vi "系统设置.vi"() -> ()   [LabVIEW 2016]
uses:
  <vilib>/Utility/miscctls.llb/LVPointTypeDef.ctl
  <userlib>/_SmartBalloon/Balloon Generic/Aesthetics.ctl
  <userlib>/_SmartBalloon/Balloon/Text Balloon.lvclass
  C:/Program Files (x86)/National Instruments/LabVIEW 2016/user.lib/_SmartBalloon/Balloon Generic/Balloon.lvclass
  <userlib>/_SmartBalloon/Balloon/Init Balloon.vi
  <vilib>/ptbypt/NI_PtbyPt.lvlib
  <vilib>/Utility/config.llb/NI_LVConfig.lvlib
  PLC/PLC.lvlib
  API/WxMessage/wxpusher.lvlib
  <userlib>/_SmartBalloon/API/SmartBalloon Library.lvclass
  <userlib>/_SmartBalloon/Balloon Generic/Balloon.lvclass
panel:
  in  "站点信息设置":bool
  in  "微信关注设置":bool
  in  "自动运行启动参数":T1
  out "一级权限":bool
  in  "定时重启配置":bool
  in  "模块启用配置":bool
  in  "短信报警设置":bool
  in  "首页显示设置":bool
  in  "跨度核查":bool
  in  "空白核查":bool
  out "选项卡控件":enum32{"自由设定", "国标协议", "流量设定"}(tab)
  in  "24H周期设置":bool[](xcontrol)
  in  "多参数运行间隔":i16=4 min=1 max=24
  in  "湿化学运行间隔":i16=4 min=1 max=24
  in  "流量阈值":dbl=4.0 min=1.0 max=24.0
  in  "时间阈值":u16=4 min=1 max=24
  in  "周期设置":enum16{"自由设定", "国标协议", "流量设定"}(ring)
  out "二级权限":bool
  in  "质控启动日期":string(combo)="关闭"
  in  "跨度核查时间":u16(ring)=6 items=["00H", "01H", "02H", "03H", "04H", "05H", "06H", "07H", "08H", "09H", "10H", "11H", "12H", "13H", "14H", "15H", "16H", "17H", "18H", "19H", "20H", "21H", "22H", "23H", "关闭"]
  in  "空白核查时间":u16(ring)=2 items=["00H", "01H", "02H", "03H", "04H", "05H", "06H", "07H", "08H", "09H", "10H", "11H", "12H", "13H", "14H", "15H", "16H", "17H", "18H", "19H", "20H", "21H", "22H", "23H", "关闭"]
  in  "输入密码":u32
  out "布尔":bool
  in  "副屏显示设置":bool
  in  "开机启动":bool caption="氨氮禁用"
  in  "运行模式":enum16{"维护模式", "常规模式", "应急模式", "质控模式"}(ring)
  # "注：周期设置分为自由设定和国标协议两种。\n1：选择自由设定情况下：运行间隔将不可选用并变灰色，周期设置可自由手动勾选\n2：选择国标协议情况下：周期时间将由运行间隔选择的时间决定，下方周期设置被禁用并无法手动勾选。\n3：选择流量设定情况下：瞬时流量连续超过流量阈值到达时间阈值设定值，仪器将自动开启测量。"
  # "质控频次："
  # "零点核查时间："
  # "跨度核查时间："
  # "启动周期设置"
  # "m3/S"
  # "秒"
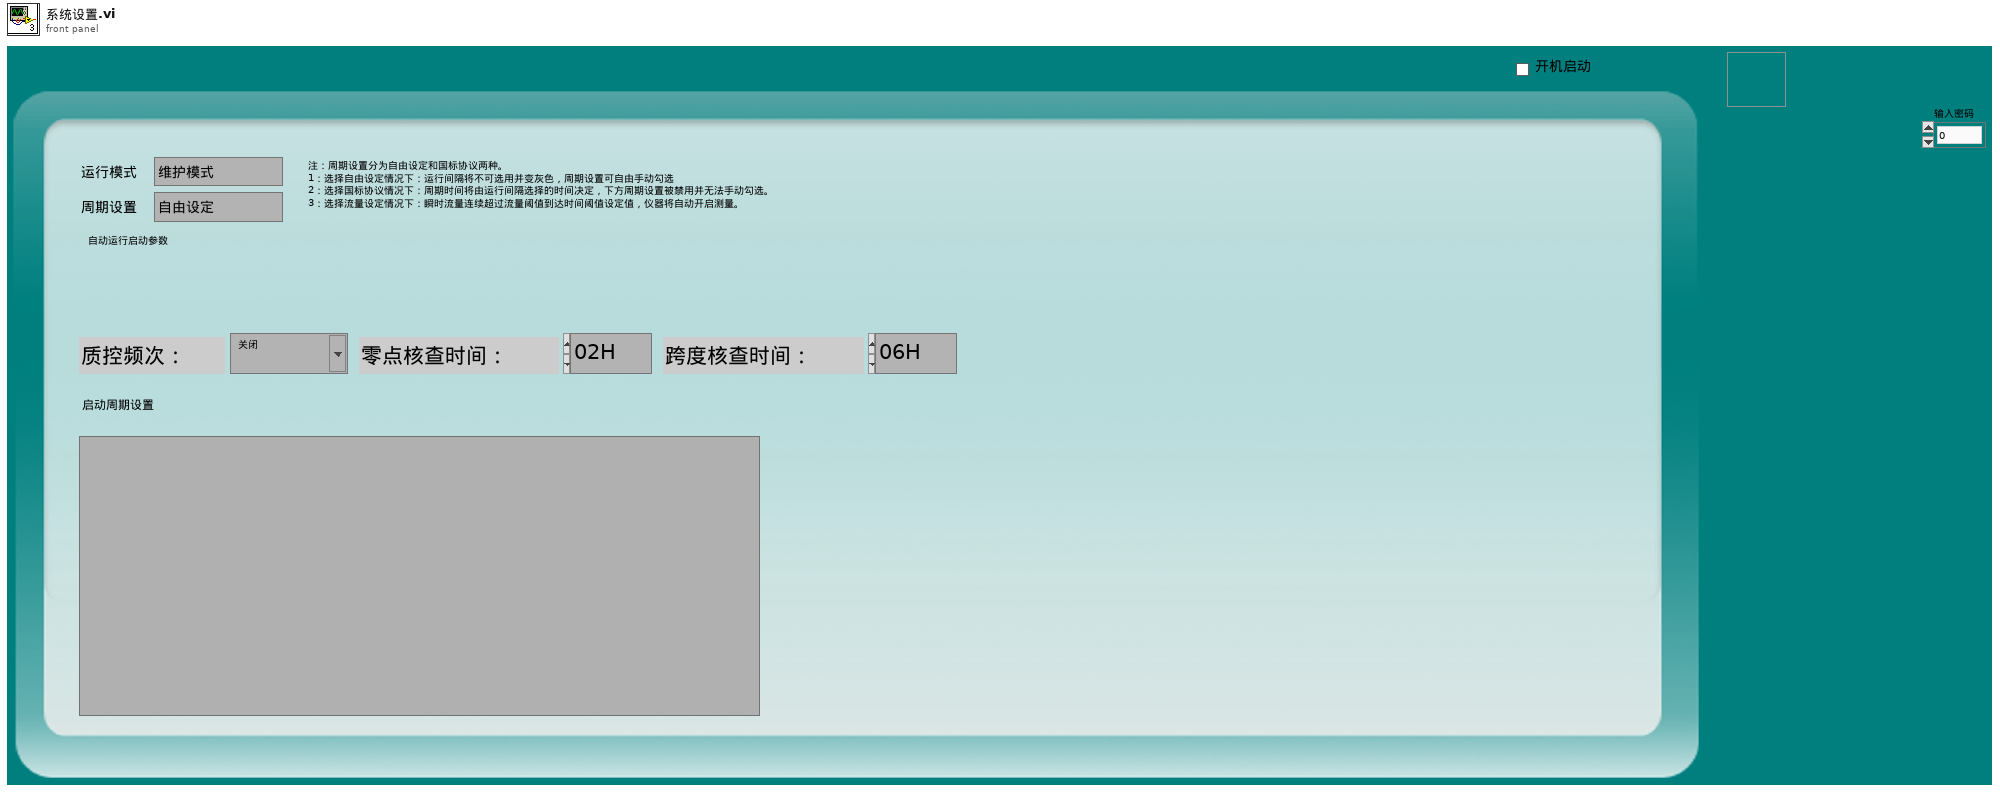
[diagram p1: front panel]
types:
  T1 = cluster{"氨氮":bool, "总磷总氮":bool, "CODmn":bool, "CODCr":bool, "多参数":bool, "超标留样启用":bool, "总氮":bool}
  T2 = typedef "LVPointTypeDef.ctl" = cluster{"Horizontal":i16, "Vertical":i16}
  T3 = cluster{"频次":enum16{"关闭", "每天", "星期一", "星期二", "星期三", "星期四", "星期五", "星期六", "星期日"}, "时":u16, "分":u16}
  T4 = typedef "LVDateTimeRec.ctl" = cluster{"秒数的小数部分":dbl, "秒":i32, "分":i32, "时":i32, "日":i32, "月":i32, "年":i32, "天数（周）":i32, "天数（年）":i32, "DST":i32}
  T5 = enum16{"关闭", "每天", "星期一", "星期二", "星期三", "星期四", "星期五", "星期六", "星期日"}
  T6 = enum32{"Bad", "Idle", "Run top level", "Running"}
  T7 = typedef "Balloon Engine.lvlib/Balloon.lvclass/Aesthetics.ctl" = cluster{"Colors":cluster{"Font Color":u32, "Panel Color":u32}, "Display Time (ms)":i32}
  T8 = typedef "NI_LVConfig.lvlib/Config Data RefNum.ctl" = refnum<k1>
  T9 = cluster{"运行模式":enum16{"维护模式", "常规模式", "应急模式", "质控模式"}}
  T10 = enum16{"启动测量", "标样核查", "零点核查", "跨度核查", "空白测试", "平行样测试", "加标回收", "空白校准", "标样校准", "初始化（清洗）", "停止测试", "仪器重启", "校时", "模式设置", "测量间隔设置"}
  T11 = cluster{"测量模式":enum16{"水样测量", "标样核查", "零点核查", "跨度核查", "空白测试", "加标回收", "平行样", "校零", "校标"}}
  T12 = cluster{"测试模式":enum16{"正常测试", "集成干预"}, "参数启用":cluster{"氨氮":bool, "总磷总氮":bool, "CODMn":bool, "CODcr":bool, "多参数":bool, "超标留样":bool, "总氮":bool}}
  T13 = cluster{"运行模式":enum16{"维护模式", "常规模式", "应急模式", "质控模式"}, "质控频次":enum16{"关闭", "每天", "星期一", "星期二", "星期三", "星期四", "星期五", "星期六", "星期日"}, "空白核查时间":u16, "跨度核查时间":u16, "24H周期设置":bool[]}
  T14 = enum32{"Invalid", "Standard", "Closed", "Hidden", "Minimized", "Maximized"}
  T15 = cluster{"氨氮":bool, "总磷总氮":bool, "CODmn":bool, "CODCr":bool, "多参数":bool, "超标留样":bool, "总氮":bool}
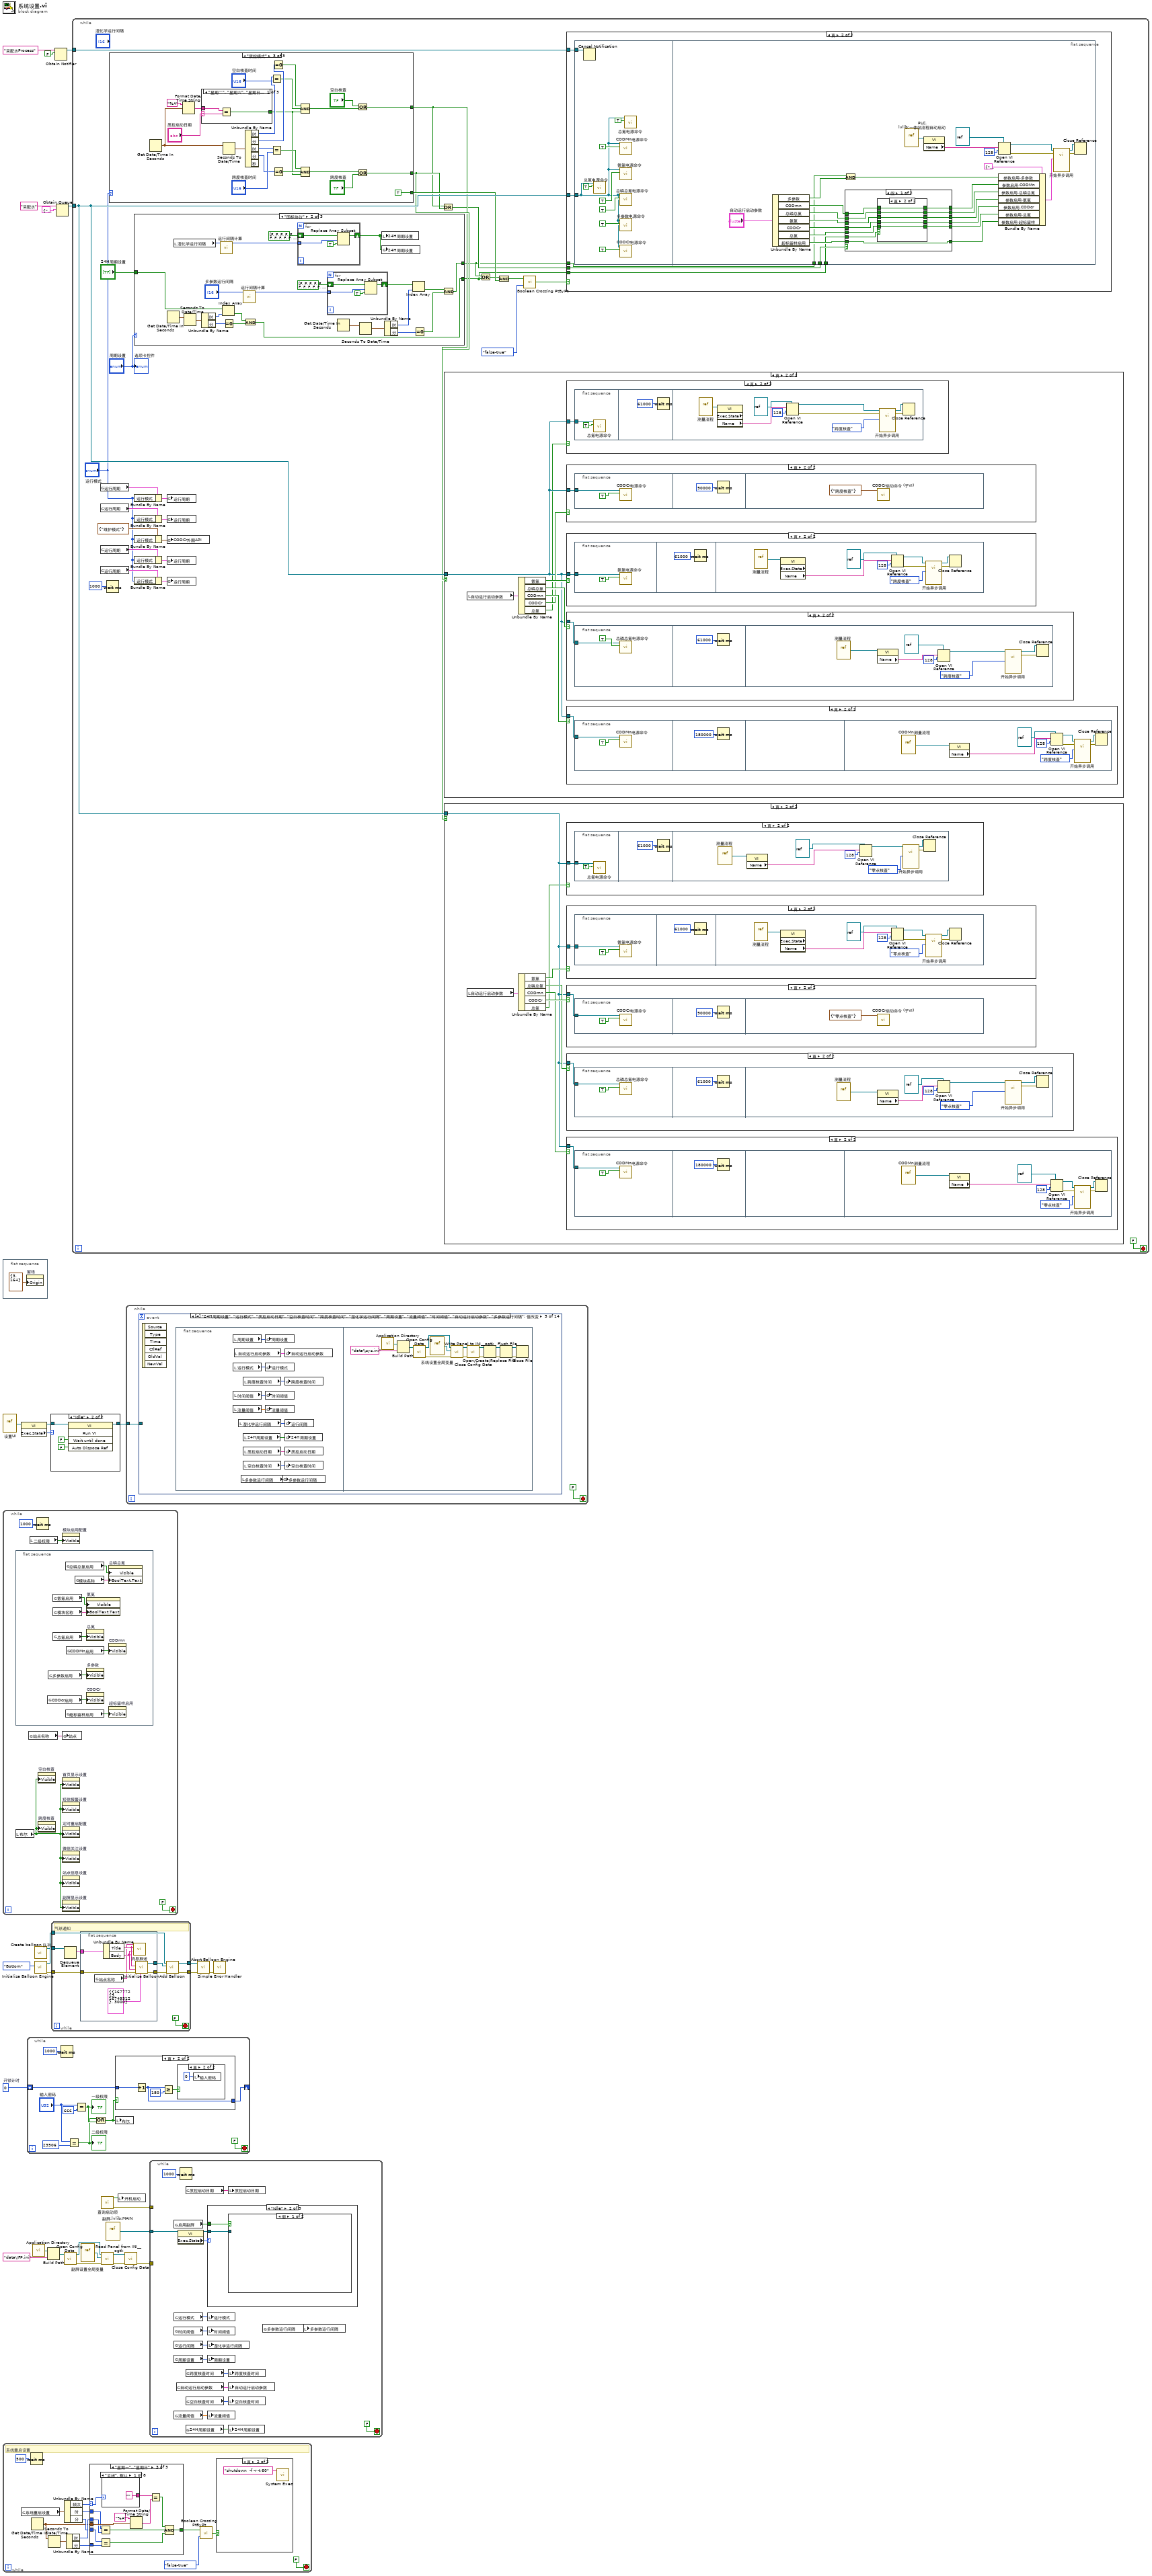
[diagram p0: block diagram]
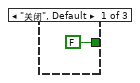
[diagram p3: hidden frame]
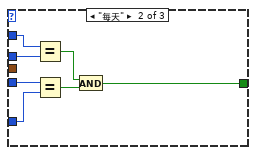
[diagram p4: hidden frame]
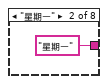
[diagram p5: hidden frame]
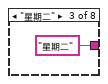
[diagram p6: hidden frame]
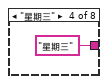
[diagram p7: hidden frame]
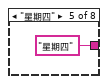
[diagram p8: hidden frame]
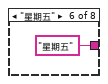
[diagram p9: hidden frame]
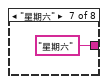
[diagram p10: hidden frame]
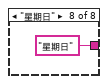
[diagram p11: hidden frame]
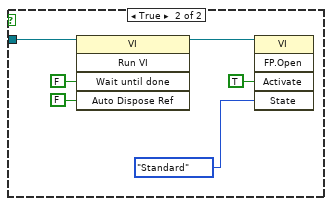
[diagram p16: hidden frame]
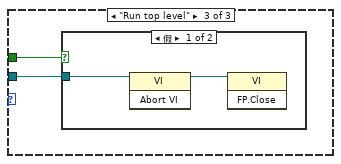
[diagram p17: hidden frame]
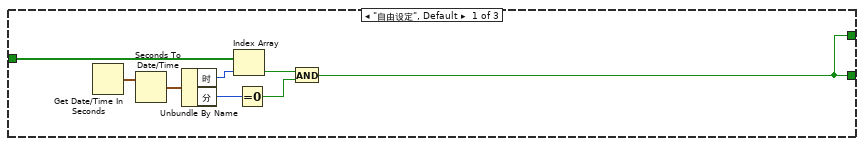
[diagram p19: hidden frame]
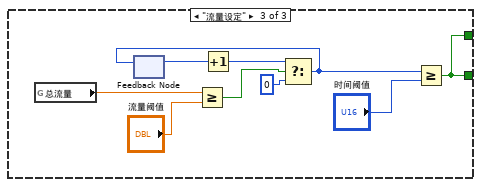
[diagram p20: hidden frame]
diagram:
  w26 = u32 0  # 开锁计时
  n1 = flat-sequence {
    frame #0 {
      n2 = property on="窗格" class="Pane"("Origin"=T2 {"Horizontal"=3, "Vertical"=164} ("原点")) -> ()  [unwired: 2 in, 2 out]
    }
  }
  n3 = vi-ref "设置UI.vi"() -> (w21:refnum<vi>)
  n4 = while {
    stop <- FALSE stop-if-true
    n5 = flat-sequence {
      frame #0 {
        n6 = global read "系统设置全局变量.vi" "CODcr启用"() -> (w45:bool)
        n7 = global read "系统设置全局变量.vi" "多参数启用"() -> (w42:bool)
        n8 = global read "系统设置全局变量.vi" "氨氮启用"() -> (w43:bool)
        n9 = global read "VAR总磷总氮全局变量.vi" "模块名称"() -> (w38:string)
        n10 = global read "系统设置全局变量.vi" "总氮启用"() -> (w39:bool)
        n11 = global read "系统设置全局变量.vi" "总磷总氮启用"() -> (w41:bool)
        n12 = global read "系统设置全局变量.vi" "超标留样启用"() -> (w40:bool)
        n13 = global read "系统设置全局变量.vi" "CODMn启用"() -> (w44:bool)
        n14 = global read "VAR总磷总氮全局变量.vi" "模块名称"() -> (w37:string)
        n15 = property on="氨氮" class="Bool (严格)"("Visible"=w43, "BoolText.Text"=w38) -> ()  [unwired: 2 in, 2 out]
        n16 = property on="总氮" class="Bool (严格)"("Visible"=w39) -> ()  [unwired: 2 in, 2 out]
        n17 = property on="多参数" class="Bool (严格)"("Visible"=w42) -> ()  [unwired: 2 in, 2 out]
        n18 = property on="CODCr" class="Bool (严格)"("Visible"=w45) -> ()  [unwired: 2 in, 2 out]
        n19 = property on="总磷总氮" class="Bool (严格)"("Visible"=w41, "BoolText.Text"=w37) -> ()  [unwired: 2 in, 2 out]
        n20 = property on="CODmn" class="Bool (严格)"("Visible"=w44) -> ()  [unwired: 2 in, 2 out]
        n21 = property on="超标留样启用" class="Bool (严格)"("Visible"=w40) -> ()  [unwired: 2 in, 2 out]
      }
    }
    n22 = local read "布尔"() -> (w33:bool)
    n23 = global read "系统设置全局变量.vi" "站点名称"() -> (w32:string)
    n24 = local read "二级权限"() -> (w34:bool)
    n25 = Wait (ms)(milliseconds to wait=u32 1000 ("等待时间（毫秒）")) -> ()  [unwired: 1 out]
    n26 = property on="空白核查" class="Bool"("Visible"=w33) -> ()  [unwired: 2 in, 2 out]
    n27 = property on="跨度核查" class="Bool"("Visible"=w33) -> ()  [unwired: 2 in, 2 out]
    n28 = property on="模块启用配置" class="Bool"("Visible"=w34) -> ()  [unwired: 2 in, 2 out]
    n29 = global write "短信服务全局变量.vi" "站点"(w32) -> ()
    n30 = property on="首页显示设置" class="Bool"("Visible"=w33) -> ()  [unwired: 2 in, 2 out]
    n31 = property on="短信报警设置" class="Bool"("Visible"=w33) -> ()  [unwired: 2 in, 2 out]
    n32 = property on="定时重启配置" class="Bool"("Visible"=w33) -> ()  [unwired: 2 in, 2 out]
    n33 = property on="微信关注设置" class="Bool"("Visible"=w33) -> ()  [unwired: 2 in, 2 out]
    n34 = property on="站点信息设置" class="Bool"("Visible"=w33) -> ()  [unwired: 2 in, 2 out]
    n35 = property on="副屏显示设置" class="Bool"("Visible"=w33) -> ()  [unwired: 2 in, 2 out]
  }
  n36 = while {
    stop <- FALSE stop-if-true
    # "系统重启设置"
    n37 = global read "系统设置全局变量.vi" "系统重启设置"() -> (w58:T3)
    n38 = Wait (ms)(milliseconds to wait=u32 500 ("等待时间（毫秒）")) -> ()  [unwired: 1 out]
    n39 = Get Date/Time In Seconds() -> (seconds since 1Jan1904=w49:timestamp)
    n40 = Seconds To Date/Time(time stamp (now)=w49) -> (date time rec=w56:T4)  [unwired: 1 in]
    n41 = Unbundle By Name(w58) -> ("频次"=w57:T5, "时"=w53:u16, "分"=w52:u16)
    n42 = Unbundle By Name(w56) -> ("时"=w55:i32, "分"=w54:i32)
    n43 = case shown="\"星期一\"..\"星期日\"" w57 {
      selector: w57 -> [_ _ w78]
      tunnel: [FALSE w61 w68] -> w48
      tunnel: w55 -> [_ w67 w72]
      tunnel: w54 -> [_ w64 w70]
      tunnel: w53 -> [_ w66 w73]
      tunnel: w52 -> [_ w65 w71]
      tunnel: w49 -> [_ _ w79]
      frame "关闭", Default {
      }
      frame "每天" {
        n44 = Equal?(x=w66, y=w67) -> (x = y?=w62:bool)
        n45 = Equal?(x=w65, y=w64) -> (x = y?=w63:bool)
        n46 = And(x=w62, y=w63) -> (x .and. y?=w61:bool)
      }
      frame "星期一".."星期日" {
        n47 = Equal?(x=w73, y=w72) -> (x = y?=w74:bool)
        n48 = Equal?(x=w71, y=w70) -> (x = y?=w75:bool)
        n49 = case shown="\"关闭\", 默认" w78 {
          tunnel: ["" ("时间格式字符串(%c)") "星期一" ("时间格式字符串(%c)") "星期二" ("时间格式字符串(%c)") "星期三" ("时间格式字符串(%c)") "星期四" ("时间格式字符串(%c)") "星期五" ("时间格式字符串(%c)") "星期六" ("时间格式字符串(%c)") "星期日" ("时间格式字符串(%c)")] -> w76
          frame "关闭", Default {
          }
          frame "星期一" {
          }
          frame "星期二" {
          }
          frame "星期三" {
          }
          frame "星期四" {
          }
          frame "星期五" {
          }
          frame "星期六" {
          }
          frame "星期日" {
          }
        }
        n50 = Format Date/Time String(time format string (%c)="%A" ("时间格式字符串(%c)"), seconds (now)=w79) -> (date/time string=w77:string)  [unwired: 1 in]
        n51 = Equal?(x=w76, y=w77) -> (x = y?=w69:bool)
        n52 = Compound Arithmetic op=AND ("复合运算")(w69, w74, w75) -> (w68:bool)
      }
    }
    n53 = call <vilib>:"Boolean Crossing PtByPt.vi"("direction"=enum16{"either", "false-true", "true-false"}."false-true", "input"=w48) -> ("crossing"=w46:bool)  [unwired: 1 in]
    n54 = case shown="真" w46 {
      frame False {
      }
      frame True {
        n55 = call <vilib>:"System Exec.vi"("command line"="shutdown  -f -r -t 60") -> ()  [unwired: 7 in, 4 out]
      }
    }
  }
  n56 = property class="VI"(reference=w21) -> (reference out=w19:refnum<vi>, "Exec.State"=w20:T6)  [unwired: 1 in, 1 out]
  n57 = while {
    shift-right: [w94] -> _
    shift-left: w26 -> [w95]
    stop <- FALSE stop-if-true
    n58 = Wait (ms)(milliseconds to wait=u32 1000 ("等待时间（毫秒）")) -> ()  [unwired: 1 out]
    n59 = Equal?(x="输入密码", y=u32 23506) -> (x = y?=w90:bool)
    "二级权限" <- w90
    n60 = Equal?(x="输入密码", y=u32 666) -> (x = y?=w91:bool)
    "一级权限" <- w91
    n61 = Or(x=w90, y=w91) -> (x .or. y?=w89:bool)
    n62 = case shown="真" w89 {
      tunnel: w95 -> [_ w102]
      tunnel: [_ w101] -> w94
      frame False {
      }
      frame True {
        n63 = Increment(x=w102) -> (x+1=w101:u32)
        n64 = Greater Or Equal?(x=w101, y=u32 180) -> (x >= y?=w99:bool)
        n65 = case shown="真" w99 {
          frame False {
          }
          frame True {
            n66 = local write "输入密码"(u32 0 ("输入密码")) -> ()
          }
        }
      }
    }
    n67 = local write "布尔"(w89) -> ()
  }
  n68 = call <vilib>:"Application Directory.vi"() -> ("Application Directory"=w8:path)
  n69 = call "Create balloon 队列.vi"() -> ("队列输出"=w1:refnum<queue>)  [unwired: 11 in]
  n70 = call <userlib>:"Initialize Balloon Engine.vi"("Balloon Direction"=enum16{"Top", "Bottom"}."Bottom" ("Balloon Position")) -> ("error out"=w3:errorcluster, "SmartBalloon Library.lvclass"=w6:refnum<class "SmartBalloon Library.lvclass">)  [unwired: 9 in]
  n71 = Build Path(base path=w8, name or relative path="data\\FP.ini" ("名称或相对路径")) -> (appended path=w15:path)
  n72 = case shown="\"Idle\"" w20 {
    tunnel: w19 -> [w104 w108]
    tunnel: [w104 w107] -> w18
    frame "Bad", Default {
    }
    frame "Idle" {
      n73 = invoke class="VI" method="Run VI"(reference=w108, "Wait until done"=FALSE ("结束前等待"), "Auto Dispose Ref"=FALSE ("自动销毁引用")) -> (reference out=w107:refnum<vi>)  [unwired: 2 in, 4 out]
    }
  }
  n74 = while {
    tunnel: w6 -> [w117]
    tunnel: [w116] -> w5
    tunnel: [w114] -> w4
    tunnel: w3 -> [w115]
    tunnel: w1 -> [w109]
    stop <- FALSE stop-if-true
    # "气球通知"
    n75 = Dequeue Element(queue=w109) -> (element=w110:cluster{"Title":string, "Body":string})  [unwired: 2 in, 3 out]
    n76 = flat-sequence {
      tunnel: w115 -> [w125]
      tunnel: [w124] -> w112
      tunnel: [w122] -> w111
      tunnel: w110 -> [w121]
      frame #0 {
        n77 = global read "系统设置全局变量.vi" "站点名称"() -> (w118:string)
        n78 = Unbundle By Name(w121) -> ("Title"=w120:string, "Body"=w119:string)
        n79 = call "消息推送.vi"("分析"=w119, "内容"=w120, "站点"=w118) -> ()  [unwired: 8 in, 1 out]
        n80 = call-poly <userlib>:"Initialize Balloon.vi"("Aesthetics"=T7 {"Colors"={"Font Color"=16777215, "Panel Color"=16749312}, "Display Time (ms)"=3000}, "error in (no error)"=w125, "Body"=w119, "Title"=w120) -> ("error out"=w122:errorcluster, "Balloon out"=w124:refnum<class "Text Balloon.lvclass">)  [unwired: 6 in]
      }
    }
    n81 = call <userlib>:"Add Balloon.vi"("error in (no error)"=w111, "Next Balloon"=w112, "SmartBalloon Engine Reference"=w117) -> ("error out"=w114:errorcluster, "SmartBalloon Engine Reference out"=w116:refnum<class "SmartBalloon Library.lvclass">)  [unwired: 7 in]
  }
  n82 = Obtain Notifier(name (unnamed)="采配水Process" ("名称（未命名）"), notification data type=FALSE) -> (notifier out=w28:refnum<notifier>)  [unwired: 2 in, 2 out]
  n83 = Obtain Queue(name (unnamed)="采配水" ("名称（未命名）"), element data type=cluster{"命令":string, "数据":variant} {"命令"="", "数据"=variant}) -> (queue out=w23:refnum<queue>)  [unwired: 3 in, 2 out]
  n84 = call <vilib>:"Open Config Data.vi"("configuration file path"=w15) -> ("error out"=w14:errorcluster, "refnum"=w11:T8)  [unwired: 8 in, 1 out]
  n85 = while {
    tunnel: w28 -> [w150]
    tunnel: w23 -> [w146]
    stop <- FALSE stop-if-true
    n86 = global read "总磷总氮断电保存全局变量.vi" "运行周期"() -> (w135:T13)
    n87 = global read "CODMn断电保存全局变量.vi" "运行周期"() -> (w133:T13)
    n88 = global read "总磷总氮断电保存全局变量.vi" "运行周期"() -> (w137:T13)
    n89 = global read "总磷总氮断电保存全局变量.vi" "运行周期"() -> (w131:T13)
    n90 = Wait (ms)(milliseconds to wait=u32 1000 ("等待时间（毫秒）")) -> ()  [unwired: 1 out]
    n91 = case shown="\"质控模式\"" "运行模式" {
      tunnel: [_ _ w386] -> w140
      tunnel: [_ _ w390] -> w139
      tunnel: [_ TRUE TRUE] -> w143
      frame "维护模式", Default {
      }
      frame "常规模式" {
      }
      frame "质控模式" {
        n92 = Get Date/Time In Seconds() -> (seconds since 1Jan1904=w395:timestamp)
        n93 = Format Date/Time String(time format string (%c)="%A" ("时间格式字符串(%c)"), seconds (now)=w395) -> (date/time string=w393:string)  [unwired: 1 in]
        n94 = case shown="\"星期二\", \"星期六\", \"星期日\", \"星期三\", \"星期四\", \"星期五\", \"星期一\"" "质控启动日期" {
          selector: "质控启动日期" -> [w411 _ _]
          tunnel: [w410 TRUE FALSE] -> w396
          tunnel: w393 -> [w409 _ _]
          frame "星期二", "星期六", "星期日", "星期三", "星期四", "星期五", "星期一" {
            n95 = Equal?(x=w409, y=w411) -> (x = y?=w410:bool)
          }
          frame "每天" {
          }
          frame "关闭", Default {
          }
        }
        n96 = Seconds To Date/Time(time stamp (now)=w395) -> (date time rec=w408:T4)  [unwired: 1 in]
        n97 = Unbundle By Name(w408) -> ("时"=w407:i32, "分"=w405:i32, "时"=w401:i32, "分"=w400:i32)  [unwired: 1 out]
        n98 = Equal?(x=w407, y="空白核查时间") -> (x = y?=w404:bool)
        n99 = Equal?(x=w401, y="跨度核查时间") -> (x = y?=w399:bool)
        n100 = Equal To 0?(x=w405) -> (x = 0?=w403:bool)
        n101 = Equal To 0?(x=w400) -> (x = 0?=w398:bool)
        n102 = Compound Arithmetic op=AND ("复合运算")(w403, w404, w396) -> (w391:bool)
        n103 = Compound Arithmetic op=AND ("复合运算")(w399, w398, w396) -> (w388:bool)
        n104 = Or(x="空白核查", y=w391) -> (x .or. y?=w390:bool)
        n105 = Or(x=w388, y="跨度核查") -> (x .or. y?=w386:bool)
      }
    }
    n106 = case shown="\"国标协议\"" "周期设置" {
      tunnel: [w153 w172 w192] -> w126
      tunnel: "24H周期设置" -> [w154 w173 _]
      tunnel: [w153 w161 w192] -> w127
      frame "自由设定", Default {
        n107 = Get Date/Time In Seconds() -> (seconds since 1Jan1904=w155:timestamp)
        n108 = Seconds To Date/Time(time stamp (now)=w155) -> (date time rec=w156:T4)  [unwired: 1 in]
        n109 = Unbundle By Name(w156) -> ("时"=w159:i32, "分"=w157:i32)
        n110 = Index Array(array=w154, index=w159) -> (element=w160:bool)
        n111 = Equal To 0?(x=w157) -> (x = 0?=w158:bool)
        n112 = And(x=w160, y=w158) -> (x .and. y?=w153:bool)
      }
      frame "国标协议" {
        n113 = Get Date/Time In Seconds() -> (seconds since 1Jan1904=w174:timestamp)
        n114 = local read "湿化学运行间隔"() -> (w183:i16)
        n115 = Seconds To Date/Time(time stamp (now)=w174) -> (date time rec=w175:T4)  [unwired: 1 in]
        n116 = Unbundle By Name(w175) -> ("时"=w178:i32, "分"=w176:i32)
        n117 = call "运行间隔计算.vi"("运行周期"=w183) -> ("数组"=w182:i32[])  [unwired: 10 in]
        n118 = Index Array(array=w173, index=w178) -> (element=w179:bool)
        n119 = Equal To 0?(x=w176) -> (x = 0?=w177:bool)
        n120 = call "运行间隔计算.vi"("运行周期"="多参数运行间隔") -> ("数组"=w164:i32[])  [unwired: 10 in]
        n121 = And(x=w179, y=w177) -> (x .and. y?=w172:bool)
        n122 = for {
          tunnel: w182 -> [w190] mode=indexing
          shift-right: [w188] -> w180
          shift-left: bool[] [FALSE, FALSE, FALSE, FALSE, FALSE, FALSE, FALSE, FALSE, FALSE, FALSE, FALSE, FALSE, FALSE, FALSE, FALSE, FALSE, FALSE, FALSE, FALSE, FALSE, FALSE, FALSE, FALSE, FALSE] ("24H周期设置") -> [w191]
          n123 = Replace Array Subset(array=w191, new element=TRUE ("新元素/子数组"), index=w190) -> (w188:bool[])
        }
        n124 = for {
          tunnel: w164 -> [w186] mode=indexing
          shift-right: [w184] -> w163
          shift-left: bool[] [FALSE, FALSE, FALSE, FALSE, FALSE, FALSE, FALSE, FALSE, FALSE, FALSE, FALSE, FALSE, FALSE, FALSE, FALSE, FALSE, FALSE, FALSE, FALSE, FALSE, FALSE, FALSE, FALSE, FALSE] ("24H周期设置") -> [w187]
          n125 = Replace Array Subset(array=w187, new element=TRUE ("新元素/子数组"), index=w186) -> (w184:bool[])
        }
        n126 = Get Date/Time In Seconds() -> (seconds since 1Jan1904=w171:timestamp)
        n127 = Seconds To Date/Time(time stamp (now)=w171) -> (date time rec=w170:T4)  [unwired: 1 in]
        n128 = local write "24H周期设置"(w180) -> ()
        n129 = global write "系统设置全局变量.vi" "24H周期设置"(w180) -> ()
        n130 = Unbundle By Name(w170) -> ("时"=w167:i32, "分"=w169:i32)
        n131 = Index Array(array=w163, index=w167) -> (element=w166:bool)
        n132 = Equal To 0?(x=w169) -> (x = 0?=w168:bool)
        n133 = And(x=w166, y=w168) -> (x .and. y?=w161:bool)
      }
      frame "流量设定" {
        n134 = global read "流量计全局变量.vi" "总流量"() -> (w200:dbl)
        n135 = feedback #1() -> (w197:i16)  [unwired: 1 in]
        n136 = Greater Or Equal?(x=w200, y="流量阈值") -> (x >= y?=w195:bool)
        n137 = Increment(x=w197) -> (x+1=w196:i16)
        n138 = Select(t=w196, s=w195, f=i16 0) -> (s? t:f=w194:i16)
        n139 = feedback-in #1(w194) -> ()
        n140 = Greater Or Equal?(x=w194, y="时间阈值") -> (x >= y?=w192:bool)
      }
    }
    n141 = Bundle By Name(cluster=w135, "运行模式"="运行模式") -> (w134:T13)
    n142 = Bundle By Name(cluster=w133, "运行模式"="运行模式") -> (w132:T13)
    n143 = Bundle By Name(cluster=T9 {"运行模式"=enum."维护模式"} ("外围API"), "运行模式"="运行模式") -> (w141:T9)
    n144 = Bundle By Name(cluster=w137, "运行模式"="运行模式") -> (w136:T13)
    n145 = Bundle By Name(cluster=w131, "运行模式"="运行模式") -> (w130:T13)
    n146 = global write "总磷总氮断电保存全局变量.vi" "运行周期"(w134) -> ()
    n147 = global write "CODMn断电保存全局变量.vi" "运行周期"(w132) -> ()
    n148 = global write "CODCr外部API.vi" "CODCr外围API"(w141) -> ()
    n149 = global write "总磷总氮断电保存全局变量.vi" "运行周期"(w136) -> ()
    n150 = global write "总磷总氮断电保存全局变量.vi" "运行周期"(w130) -> ()
    n151 = Or(x=w139, y=w140) -> (x .or. y?=w138:bool)
    n152 = case shown="真" w140 {
      tunnel: w146 -> [_ w202]
      frame False {
      }
      frame True {
        n153 = local read "自动运行启动参数"() -> (w207:T1)
        n154 = Unbundle By Name(w207) -> ("氨氮"=w206:bool, "总磷总氮"=w205:bool, "CODmn"=w204:bool, "CODCr"=w203:bool, "总氮"=w201:bool)
        n155 = case shown="真" w201 {
          tunnel: w202 -> [_ w208]
          frame False {
          }
          frame True {
            n156 = flat-sequence {
              tunnel: w208 -> [w210]
              frame #0 {
                n157 = call "总氮电源命令.vi"("通电/断电"=TRUE, "队列"=w210) -> ()  [unwired: 9 in, 1 out]
              }
              frame #1 {
                n158 = Wait (ms)(milliseconds to wait=u32 61000 ("等待时间（毫秒）")) -> ()  [unwired: 1 out]
              }
              frame #2 {
                n159 = vi-ref "测量流程.vi"() -> (w220:refnum<vi>)
                n160 = property class="VI" props=["Exec.State", "Name"](reference=w220) -> ("Name"=w219:string)  [unwired: 1 in, 3 out]
                n161 = Open VI Reference(type specifier VI Refnum (for type only)=refnum<vi> refnum, vi path=w219, options=128 ("选项")) -> (vi reference=w214:refnum<vi>, error out=w216:errorcluster)  [unwired: 3 in]
                n162 = call-by-ref "开始异步调用"(reference=w214, error in=w216, "控制命令"=T10."跨度核查") -> (reference out=w217:refnum<vi>, error out=w218:errorcluster)  [unwired: 11 in]
                n163 = Close Reference(reference=w217, error in (no error)=w218) -> ()  [unwired: 1 out]
              }
            }
          }
        }
        n164 = case shown="真" w203 {
          tunnel: w202 -> [_ w221]
          frame False {
          }
          frame True {
            n165 = flat-sequence {
              tunnel: w221 -> [w222]
              frame #0 {
                n166 = call "CODCr电源命令.vi"("通电/断电"=TRUE, "队列"=w222) -> ()  [unwired: 9 in, 1 out]
              }
              frame #1 {
                n167 = Wait (ms)(milliseconds to wait=u32 90000 ("等待时间（毫秒）")) -> ()  [unwired: 1 out]
              }
              frame #2 {
                n168 = call "CODCr启动命令 (子VI).vi"("启动测量模式"=T11 {"测量模式"=enum."跨度核查"}) -> ()  [unwired: 11 in]
              }
            }
          }
        }
        n169 = case shown="真" w206 {
          tunnel: w202 -> [_ w251]
          frame False {
          }
          frame True {
            n170 = flat-sequence {
              tunnel: w251 -> [w252]
              frame #0 {
                n171 = call "氨氮电源命令.vi"("通电/断电"=TRUE, "队列"=w252) -> ()  [unwired: 9 in, 1 out]
              }
              frame #1 {
                n172 = Wait (ms)(milliseconds to wait=u32 61000 ("等待时间（毫秒）")) -> ()  [unwired: 1 out]
              }
              frame #2 {
                n173 = vi-ref "测量流程.vi"() -> (w263:refnum<vi>)
                n174 = property class="VI" props=["Exec.State", "Name"](reference=w263) -> ("Name"=w262:string)  [unwired: 1 in, 3 out]
                n175 = Open VI Reference(type specifier VI Refnum (for type only)=refnum<vi> refnum, vi path=w262, options=128 ("选项")) -> (vi reference=w257:refnum<vi>, error out=w259:errorcluster)  [unwired: 3 in]
                n176 = call-by-ref "开始异步调用"(reference=w257, error in=w259, "控制命令"=T10."跨度核查") -> (reference out=w260:refnum<vi>, error out=w261:errorcluster)  [unwired: 11 in]
                n177 = Close Reference(reference=w260, error in (no error)=w261) -> ()  [unwired: 1 out]
              }
            }
          }
        }
        n178 = case shown="真" w205 {
          tunnel: w202 -> [_ w239]
          frame False {
          }
          frame True {
            n179 = flat-sequence {
              tunnel: w239 -> [w240]
              frame #0 {
                n180 = call "总磷总氮电源命令.vi"("通电/断电"=TRUE, "队列"=w240) -> ()  [unwired: 9 in, 1 out]
              }
              frame #1 {
                n181 = Wait (ms)(milliseconds to wait=u32 61000 ("等待时间（毫秒）")) -> ()  [unwired: 1 out]
              }
              frame #2 {
                n182 = vi-ref "测量流程.vi"() -> (w248:refnum<vi>)
                n183 = property class="VI"(reference=w248) -> ("Name"=w249:string)  [unwired: 1 in, 2 out]
                n184 = Open VI Reference(type specifier VI Refnum (for type only)=refnum<vi> refnum, vi path=w249, options=128 ("选项")) -> (vi reference=w247:refnum<vi>)  [unwired: 3 in, 1 out]
                n185 = call-by-ref "开始异步调用"(reference=w247, "控制命令"=T10."跨度核查") -> (reference out=w246:refnum<vi>, error out=w245:errorcluster)  [unwired: 12 in]
                n186 = Close Reference(reference=w246, error in (no error)=w245) -> ()  [unwired: 1 out]
              }
            }
          }
        }
        n187 = case shown="真" w204 {
          tunnel: w202 -> [_ w226]
          frame False {
          }
          frame True {
            n188 = flat-sequence {
              tunnel: w226 -> [w227]
              frame #0 {
                n189 = call "CODMn电源命令.vi"("通电/断电"=TRUE, "队列"=w227) -> ()  [unwired: 9 in, 1 out]
              }
              frame #1 {
                n190 = Wait (ms)(milliseconds to wait=u32 180000 ("等待时间（毫秒）")) -> ()  [unwired: 1 out]
              }
              frame #2 {
              }
              frame #3 {
                n191 = vi-ref "CODMn测量流程.vi"() -> (w237:refnum<vi>)
                n192 = property class="VI"(reference=w237) -> ("Name"=w238:string)  [unwired: 1 in, 2 out]
                n193 = Open VI Reference(type specifier VI Refnum (for type only)=refnum<vi> refnum, vi path=w238, options=128 ("选项")) -> (vi reference=w232:refnum<vi>, error out=w234:errorcluster)  [unwired: 3 in]
                n194 = call-by-ref "开始异步调用"(reference=w232, error in=w234, "控制命令"=T10."跨度核查") -> (reference out=w235:refnum<vi>, error out=w236:errorcluster)  [unwired: 11 in]
                n195 = Close Reference(reference=w235, error in (no error)=w236) -> ()  [unwired: 1 out]
              }
            }
          }
        }
      }
    }
    n196 = case shown="真" w139 {
      tunnel: w146 -> [_ w265]
      frame False {
      }
      frame True {
        n197 = local read "自动运行启动参数"() -> (w270:T1)
        n198 = Unbundle By Name(w270) -> ("氨氮"=w269:bool, "总磷总氮"=w266:bool, "CODmn"=w267:bool, "CODCr"=w268:bool, "总氮"=w264:bool)
        n199 = case shown="真" w264 {
          tunnel: w265 -> [_ w271]
          frame False {
          }
          frame True {
            n200 = flat-sequence {
              tunnel: w271 -> [w273]
              frame #0 {
                n201 = call "总氮电源命令.vi"("通电/断电"=TRUE, "队列"=w273) -> ()  [unwired: 9 in, 1 out]
              }
              frame #1 {
                n202 = Wait (ms)(milliseconds to wait=u32 61000 ("等待时间（毫秒）")) -> ()  [unwired: 1 out]
              }
              frame #2 {
                n203 = vi-ref "测量流程.vi"() -> (w280:refnum<vi>)
                n204 = property class="VI"(reference=w280) -> ("Name"=w281:string)  [unwired: 1 in, 2 out]
                n205 = Open VI Reference(type specifier VI Refnum (for type only)=refnum<vi> refnum, vi path=w281, options=128 ("选项")) -> (vi reference=w279:refnum<vi>)  [unwired: 3 in, 1 out]
                n206 = call-by-ref "开始异步调用"(reference=w279, "控制命令"=T10."零点核查") -> (reference out=w278:refnum<vi>, error out=w277:errorcluster)  [unwired: 12 in]
                n207 = Close Reference(reference=w278, error in (no error)=w277) -> ()  [unwired: 1 out]
              }
            }
          }
        }
        n208 = case shown="真" w269 {
          tunnel: w265 -> [_ w313]
          frame False {
          }
          frame True {
            n209 = flat-sequence {
              tunnel: w313 -> [w314]
              frame #0 {
                n210 = call "氨氮电源命令.vi"("通电/断电"=TRUE, "队列"=w314) -> ()  [unwired: 9 in, 1 out]
              }
              frame #1 {
                n211 = Wait (ms)(milliseconds to wait=u32 61000 ("等待时间（毫秒）")) -> ()  [unwired: 1 out]
              }
              frame #2 {
                n212 = vi-ref "测量流程.vi"() -> (w325:refnum<vi>)
                n213 = property class="VI" props=["Exec.State", "Name"](reference=w325) -> ("Name"=w324:string)  [unwired: 1 in, 3 out]
                n214 = Open VI Reference(type specifier VI Refnum (for type only)=refnum<vi> refnum, vi path=w324, options=128 ("选项")) -> (vi reference=w319:refnum<vi>, error out=w321:errorcluster)  [unwired: 3 in]
                n215 = call-by-ref "开始异步调用"(reference=w319, error in=w321, "控制命令"=T10."零点核查") -> (reference out=w322:refnum<vi>, error out=w323:errorcluster)  [unwired: 11 in]
                n216 = Close Reference(reference=w322, error in (no error)=w323) -> ()  [unwired: 1 out]
              }
            }
          }
        }
        n217 = case shown="真" w268 {
          tunnel: w265 -> [_ w283]
          frame False {
          }
          frame True {
            n218 = flat-sequence {
              tunnel: w283 -> [w284]
              frame #0 {
                n219 = call "CODCr电源命令.vi"("通电/断电"=TRUE, "队列"=w284) -> ()  [unwired: 9 in, 1 out]
              }
              frame #1 {
                n220 = Wait (ms)(milliseconds to wait=u32 90000 ("等待时间（毫秒）")) -> ()  [unwired: 1 out]
              }
              frame #2 {
                n221 = call "CODCr启动命令 (子VI).vi"("启动测量模式"=T11 {"测量模式"=enum."零点核查"}) -> ()  [unwired: 11 in]
              }
            }
          }
        }
        n222 = case shown="真" w266 {
          tunnel: w265 -> [_ w301]
          frame False {
          }
          frame True {
            n223 = flat-sequence {
              tunnel: w301 -> [w302]
              frame #0 {
                n224 = call "总磷总氮电源命令.vi"("通电/断电"=TRUE, "队列"=w302) -> ()  [unwired: 9 in, 1 out]
              }
              frame #1 {
                n225 = Wait (ms)(milliseconds to wait=u32 61000 ("等待时间（毫秒）")) -> ()  [unwired: 1 out]
              }
              frame #2 {
                n226 = vi-ref "测量流程.vi"() -> (w310:refnum<vi>)
                n227 = property class="VI"(reference=w310) -> ("Name"=w311:string)  [unwired: 1 in, 2 out]
                n228 = Open VI Reference(type specifier VI Refnum (for type only)=refnum<vi> refnum, vi path=w311, options=128 ("选项")) -> (vi reference=w309:refnum<vi>)  [unwired: 3 in, 1 out]
                n229 = call-by-ref "开始异步调用"(reference=w309, "控制命令"=T10."零点核查") -> (reference out=w308:refnum<vi>, error out=w307:errorcluster)  [unwired: 12 in]
                n230 = Close Reference(reference=w308, error in (no error)=w307) -> ()  [unwired: 1 out]
              }
            }
          }
        }
        n231 = case shown="真" w267 {
          tunnel: w265 -> [_ w288]
          frame False {
          }
          frame True {
            n232 = flat-sequence {
              tunnel: w288 -> [w289]
              frame #0 {
                n233 = call "CODMn电源命令.vi"("通电/断电"=TRUE, "队列"=w289) -> ()  [unwired: 9 in, 1 out]
              }
              frame #1 {
                n234 = Wait (ms)(milliseconds to wait=u32 180000 ("等待时间（毫秒）")) -> ()  [unwired: 1 out]
              }
              frame #2 {
              }
              frame #3 {
                n235 = vi-ref "CODMn测量流程.vi"() -> (w299:refnum<vi>)
                n236 = property class="VI"(reference=w299) -> ("Name"=w300:string)  [unwired: 1 in, 2 out]
                n237 = Open VI Reference(type specifier VI Refnum (for type only)=refnum<vi> refnum, vi path=w300, options=128 ("选项")) -> (vi reference=w294:refnum<vi>, error out=w296:errorcluster)  [unwired: 3 in]
                n238 = call-by-ref "开始异步调用"(reference=w294, error in=w296, "控制命令"=T10."零点核查") -> (reference out=w297:refnum<vi>, error out=w298:errorcluster)  [unwired: 11 in]
                n239 = Close Reference(reference=w297, error in (no error)=w298) -> ()  [unwired: 1 out]
              }
            }
          }
        }
      }
    }
    n240 = Or(x=w127, y=w126) -> (x .or. y?=w128:bool)
    n241 = And(x=w128, y=w143) -> (x .and. y?=w142:bool)
    n242 = call <vilib>:"Boolean Crossing PtByPt.vi"("direction"=enum16{"either", "false-true", "true-false"}."false-true", "input"=w142) -> ("crossing"=w148:bool)  [unwired: 1 in]
    n243 = case shown="真" w148 {
      tunnel: w150 -> [_ w330]
      tunnel: w146 -> [_ w329]
      tunnel: w138 -> [_ w328]
      tunnel: w127 -> [_ w327]
      tunnel: w126 -> [_ w326]
      frame False {
      }
      frame True {
        n244 = flat-sequence {
          tunnel: w330 -> [w339]
          tunnel: w329 -> [w332]
          tunnel: w328 -> [w356]
          tunnel: w327 -> [w341]
          tunnel: w326 -> [w340]
          frame #0 {
            n245 = Cancel Notification(0:w339) -> ()  [unwired: 1 in, 3 out]
            n246 = call "总氮电源命令.vi"("通电/断电"=TRUE, "队列"=w332) -> ()  [unwired: 9 in, 1 out]
            n247 = call "CODMn电源命令.vi"("通电/断电"=TRUE, "队列"=w332) -> ()  [unwired: 9 in, 1 out]
            n248 = call "氨氮电源命令.vi"("通电/断电"=TRUE, "队列"=w332) -> ()  [unwired: 9 in, 1 out]
            n249 = call "总磷总氮电源命令.vi"("通电/断电"=TRUE, "队列"=w332) -> ()  [unwired: 9 in, 1 out]
            n250 = call "多参数电源命令.vi"("通电/断电"=TRUE, "队列"=w332) -> ()  [unwired: 9 in, 1 out]
            n251 = call "CODCr电源命令.vi"("通电/断电"=TRUE, "队列"=w332) -> ()  [unwired: 9 in, 1 out]
            n252 = call "总氮电源命令.vi"("通电/断电"=TRUE, "队列"=w332) -> ()  [unwired: 9 in, 1 out]
          }
          frame #1 {
            n253 = Unbundle By Name("自动运行启动参数") -> ("多参数"=w350:bool, "CODmn"=w351:bool, "总磷总氮"=w352:bool, "氨氮"=w353:bool, "CODCr"=w354:bool, "总氮"=w348:bool, "超标留样启用"=w347:bool)
            n254 = And(x=w341, y=w350) -> (x .and. y?=w342:bool)
            n255 = case shown="假" w356 {
              tunnel: [w378 _] -> w367
              tunnel: [w376 _] -> w366
              tunnel: [w372 _] -> w365
              tunnel: [w373 _] -> w364
              tunnel: w354 -> [w371 _]
              tunnel: w353 -> [w374 _]
              tunnel: w352 -> [w375 _]
              tunnel: w351 -> [w377 _]
              tunnel: [w369 _] -> w349
              tunnel: w348 -> [w370 _]
              tunnel: w347 -> [w368 _]
              tunnel: [w368 _] -> w344
              tunnel: w340 -> [w379 _]
              frame False {
                n256 = case shown="真" w379 {
                  tunnel: [_ w384] -> w378
                  tunnel: w377 -> [_ w384]
                  tunnel: [_ w383] -> w376
                  tunnel: w375 -> [_ w383]
                  tunnel: [_ w382] -> w373
                  tunnel: w374 -> [_ w382]
                  tunnel: [_ w381] -> w372
                  tunnel: w371 -> [_ w381]
                  tunnel: [_ w380] -> w369
                  tunnel: w370 -> [_ w380]
                  frame False {
                  }
                  frame True {
                  }
                }
              }
              frame True {
              }
            }
            n257 = vi-ref "PLC.lvlib:一体站流程自动启动.vi"() -> (w361:refnum<vi>)
            n258 = property class="VI"(reference=w361) -> ("Name"=w362:string)  [unwired: 1 in, 2 out]
            n259 = Bundle By Name(cluster=T12 {"测试模式"=enum."正常测试", "参数启用"={"氨氮"=FALSE, "总磷总氮"=FALSE, "CODMn"=FALSE, "CODcr"=FALSE, "多参数"=FALSE, "超标留样"=FALSE, "总氮"=FALSE}} ("参数"), "参数启用.多参数"=w342, "参数启用.CODMn"=w367, "参数启用.总磷总氮"=w366, "参数启用.氨氮"=w364, "参数启用.CODcr"=w365, "参数启用.总氮"=w349, "参数启用.超标留样"=w344) -> (w345:T12)
            n260 = Open VI Reference(type specifier VI Refnum (for type only)=refnum<vi> refnum, vi path=w362, options=128 ("选项")) -> (vi reference=w360:refnum<vi>, error out=w359:errorcluster)  [unwired: 3 in]
            n261 = call-by-ref "开始异步调用"(reference=w360, error in=w359, "参数"=w345) -> (reference out=w358:refnum<vi>, error out=w357:errorcluster)  [unwired: 11 in]
            n262 = Close Reference(reference=w358, error in (no error)=w357) -> ()  [unwired: 1 out]
          }
        }
      }
    }
    "选项卡控件" <- "周期设置"
  }
  n263 = vi-ref "副屏设置全局变量.vi"() -> (w12:refnum<vi>)
  n264 = call "查询启动项.vi"() -> ("error out"=w17:errorcluster, "包含启动项"=w27:bool)  [unwired: 10 in]
  n265 = call <userlib>:"Read Panel from INI__ogtk.vi"("error in (no error)"=w14, "VI ref"=w12, "refnum"=w11) -> ("error out"=w13:errorcluster, "refnum out"=w10:T8)  [unwired: 7 in]
  n266 = vi-ref "副屏.lvlib:MAIN.vi"() -> (w22:refnum<vi>)
  n267 = local write "开机启动"(w27) -> ()
  n268 = call <vilib>:"Close Config Data.vi"("error in (no error)"=w13, "refnum"=w10) -> ("error out"=w9:errorcluster)  [unwired: 8 in, 1 out]
  n269 = while {
    tunnel: w18 -> [w414]
    stop <- FALSE stop-if-true
    n270 = event shown="[4] \"24H周期设置\", \"运行模式\", \"质控启动日期\", \"空白核查时间\", \"跨度核查时间\", \"湿化学运行间隔\", \"周期设置\", \"流量阈值\", \"时间阈值\", \"自动运行启动参数\", \"多参数运行间隔\": 值改变" {
      selector: _ -> [_ _ _ _ _ _ _ _ _ _ _ _ _ _]
      dyn-events: _ -> [_ _ _ _ _ _ _ _ _ _ _ _ _ _]
      timeout: _ -> [_ _ _ _ _ _ _ _ _ _ _ _ _ _]
      tunnel: w414 -> [_ _ _ _ _ _ _ _ _ _ _ w462 _ _]
      event Timeout {
        n271 = event-data() -> ()  [unwired: 1 in, 3 out]
      }
      event "站点信息设置": Value Change {
        n272 = event-data() -> ()  [unwired: 1 in, 6 out]
        n273 = call "站点信息设置.vi"() -> ()  [unwired: 12 in]
      }
      event "定时重启配置": Value Change {
        n274 = event-data() -> ()  [unwired: 1 in, 6 out]
        n275 = call "重启设置.vi"() -> ()  [unwired: 12 in]
      }
      event "模块启用配置": Value Change {
        n276 = event-data() -> ()  [unwired: 1 in, 6 out]
        n277 = call "模块启用配置框.vi"() -> ()  [unwired: 12 in]
      }
      event "24H周期设置", "运行模式", "质控启动日期", "空白核查时间", "跨度核查时间", "湿化学运行间隔", "周期设置", "流量阈值", "时间阈值", "自动运行启动参数", "多参数运行间隔": Value Change {
        n278 = event-data() -> ()  [unwired: 1 in, 6 out]
        n279 = flat-sequence {
          frame #0 {
            n280 = local read "周期设置"() -> (w420:enum16{"自由设定", "国标协议", "流量设定"})
            n281 = local read "运行模式"() -> (w426:enum16{"维护模式", "常规模式", "应急模式", "质控模式"})
            n282 = local read "时间阈值"() -> (w419:u16)
            n283 = local read "流量阈值"() -> (w418:dbl)
            n284 = local read "自动运行启动参数"() -> (w417:T1)
            n285 = local read "湿化学运行间隔"() -> (w421:i16)
            n286 = local read "多参数运行间隔"() -> (w416:i16)
            n287 = local read "跨度核查时间"() -> (w422:u16)
            n288 = local read "24H周期设置"() -> (w425:bool[])
            n289 = local read "质控启动日期"() -> (w424:string)
            n290 = local read "空白核查时间"() -> (w423:u16)
            n291 = global write "系统设置全局变量.vi" "周期设置"(w420) -> ()
            n292 = global write "系统设置全局变量.vi" "运行模式"(w426) -> ()
            n293 = global write "系统设置全局变量.vi" "时间阈值"(w419) -> ()
            n294 = global write "系统设置全局变量.vi" "流量阈值"(w418) -> ()
            n295 = global write "系统设置全局变量.vi" "多参数运行间隔"(w416) -> ()
            n296 = global write "系统设置全局变量.vi" "自动运行启动参数"(w417) -> ()
            n297 = global write "系统设置全局变量.vi" "跨度核查时间"(w422) -> ()
            n298 = global write "系统设置全局变量.vi" "运行间隔"(w421) -> ()
            n299 = global write "系统设置全局变量.vi" "24H周期设置"(w425) -> ()
            n300 = global write "系统设置全局变量.vi" "质控启动日期"(w424) -> ()
            n301 = global write "系统设置全局变量.vi" "空白核查时间"(w423) -> ()
          }
          frame #1 {
            n302 = call <vilib>:"Application Directory.vi"() -> ("Application Directory"=w440:path)
            n303 = Build Path(base path=w440, name or relative path="data\\sys.ini" ("名称或相对路径")) -> (appended path=w438:path)
            n304 = call <vilib>:"Open Config Data.vi"("configuration file path"=w438) -> ("error out"=w434:errorcluster, "refnum"=w437:T8)  [unwired: 8 in, 1 out]
            n305 = vi-ref "系统设置全局变量.vi"() -> (w436:refnum<vi>)
            n306 = call <userlib>:"Write Panel to INI__ogtk.vi"("error in (no error)"=w434, "VI ref"=w436, "refnum"=w437) -> ("error out"=w433:errorcluster, "refnum out"=w435:T8)  [unwired: 7 in]
            n307 = call <vilib>:"Close Config Data.vi"("error in (no error)"=w433, "refnum"=w435) -> ("error out"=w428:errorcluster, "file path"=w427:path)  [unwired: 8 in]
            n308 = Open/Create/Replace File(file path (use dialog)=w427, error in=w428) -> (refnum out=w431:refnum<file>, error out=w432:errorcluster)  [unwired: 4 in, 1 out]
            n309 = Flush File(refnum=w431, error in=w432) -> (refnum out=w430:refnum<file>, error out=w429:errorcluster)
            n310 = Close File(refnum=w430, error in=w429) -> ()  [unwired: 2 out]
          }
        }
      }
      event "湿化学运行间隔", "多参数运行间隔": Mouse Down {
        n311 = event-data() -> ("CtlRef"=w444:refnum<vi>)  [unwired: 1 in, 7 out]
        n312 = property class="DigNum (严格)"(reference=w444) -> (reference out=w443:refnum<vi>, "Value"=w442:i16)  [unwired: 1 in, 1 out]
        n313 = call "数字键盘.vi"("OldNumber"=w442) -> ("NewNumber"=w441:sgl)
        n314 = property class="DigNum (严格)"(reference=w443, "Val(Sgnl)"=w441) -> ()  [unwired: 1 in, 2 out]
      }
      event "流量阈值": Mouse Down {
        n315 = event-data() -> ("CtlRef"=w448:refnum<vi>)  [unwired: 1 in, 7 out]
        n316 = property class="DigNum (严格)"(reference=w448) -> (reference out=w447:refnum<vi>, "Value"=w446:dbl)  [unwired: 1 in, 1 out]
        n317 = call "数字键盘.vi"("OldNumber"=w446) -> ("NewNumber"=w445:sgl)
        n318 = property class="DigNum (严格)"(reference=w447, "Val(Sgnl)"=w445) -> ()  [unwired: 1 in, 2 out]
      }
      event "时间阈值": Mouse Down {
        n319 = event-data() -> ("CtlRef"=w452:refnum<vi>)  [unwired: 1 in, 7 out]
        n320 = property class="DigNum (严格)"(reference=w452) -> (reference out=w451:refnum<vi>, "Value"=w450:u16)  [unwired: 1 in, 1 out]
        n321 = call "数字键盘.vi"("OldNumber"=w450) -> ("NewNumber"=w449:sgl)
        n322 = property class="DigNum (严格)"(reference=w451, "Val(Sgnl)"=w449) -> ()  [unwired: 1 in, 2 out]
      }
      event "开机启动": Value Change {
        n323 = event-data() -> ("NewVal"=w453:bool)  [unwired: 1 in, 5 out]
        n324 = case shown="假" w453 {
          frame False {
            n325 = call "删除启动项.vi"() -> ("删除标记"=w454:bool)  [unwired: 10 in, 1 out]
            n326 = case shown="假" w454 {
              frame False {
                n327 = local write "开机启动"(TRUE ("开机启动")) -> ()
                n328 = One Button Dialog(message="启动项删除失败" ("消息")) -> ()  [unwired: 1 in, 1 out]
              }
              frame True {
              }
            }
          }
          frame True {
            n329 = call "添加启动项.vi"() -> ("添加成功标记"=w457:bool)  [unwired: 10 in, 1 out]
            n330 = case shown="假" w457 {
              frame False {
                n331 = local write "开机启动"(FALSE ("开机启动")) -> ()
                n332 = One Button Dialog(message="启动项添加失败" ("消息")) -> ()  [unwired: 1 in, 1 out]
              }
              frame True {
              }
            }
          }
        }
      }
      event "副屏显示设置": Value Change {
        n333 = event-data() -> ()  [unwired: 1 in, 6 out]
        n334 = call "副屏设置.vi"() -> ()  [unwired: 12 in]
      }
      event "首页显示设置": Value Change {
        n335 = event-data() -> ()  [unwired: 1 in, 6 out]
        n336 = call "首页显示设置.vi"() -> ()  [unwired: 12 in]
      }
      event "短信报警设置": Value Change {
        n337 = event-data() -> ()  [unwired: 1 in, 6 out]
        n338 = invoke class="VI" method="FP.Open"(reference=w462, "Activate"=TRUE ("激活？"), "State"=T14."Standard" ("状态")) -> ()  [unwired: 2 in, 5 out]
      }
      event "布尔": Mouse Down {
        n339 = event-data() -> ("CtlRef"=w464:refnum<vi>)  [unwired: 1 in, 6 out]
        n340 = property class="Bool (严格)"(reference=w464) -> ("Value"=w463:bool)  [unwired: 1 in, 2 out]
        n341 = case shown="假" w463 {
          tunnel: [w466 _] -> w465
          frame False {
            n342 = call "数字密码键盘.vi"() -> ("NewNumber"=w466:sgl)  [unwired: 1 in]
          }
          frame True {
          }
        }
        n343 = local write "输入密码"(w465) -> ()
      }
      event "微信关注设置": Value Change {
        n344 = event-data() -> ()  [unwired: 1 in, 6 out]
        n345 = global read "短信服务全局变量.vi" "站点"() -> (w467:string)
        n346 = call "创建参数二维码.vi"("站点"=w467) -> ()  [unwired: 11 in]
      }
    }
  }
  n347 = while {
    tunnel: w22 -> [w480]
    tunnel: w17 -> [_]
    tunnel: w9 -> [_]
    stop <- FALSE stop-if-true
    n348 = global read "副屏设置全局变量.vi" "启用副屏"() -> (w478:bool)
    n349 = global read "系统设置全局变量.vi" "运行模式"() -> (w471:enum16{"维护模式", "常规模式", "应急模式", "质控模式"})
    n350 = global read "系统设置全局变量.vi" "时间阈值"() -> (w469:u16)
    n351 = global read "系统设置全局变量.vi" "运行间隔"() -> (w472:i16)
    n352 = global read "系统设置全局变量.vi" "周期设置"() -> (w473:enum16{"自由设定", "国标协议", "流量设定"})
    n353 = global read "系统设置全局变量.vi" "流量阈值"() -> (w470:dbl)
    n354 = global read "系统设置全局变量.vi" "自动运行启动参数"() -> (w481:T15)
    n355 = property class="VI"(reference=w480) -> (reference out=w477:refnum<vi>, "Exec.State"=w479:T6)  [unwired: 1 in, 1 out]
    n356 = Wait (ms)(milliseconds to wait=u32 1000 ("等待时间（毫秒）")) -> ()  [unwired: 1 out]
    n357 = global read "系统设置全局变量.vi" "质控启动日期"() -> (w476:string)
    n358 = global read "系统设置全局变量.vi" "跨度核查时间"() -> (w474:u16)
    n359 = global read "系统设置全局变量.vi" "空白核查时间"() -> (w475:u16)
    n360 = global read "系统设置全局变量.vi" "24H周期设置"() -> (w482:bool[])
    n361 = case shown="\"Idle\"" w479 {
      tunnel: w478 -> [_ w485 w493]
      tunnel: w477 -> [_ w486 w494]
      frame "Bad", Default {
      }
      frame "Idle" {
        n362 = case shown="假" w485 {
          tunnel: w486 -> [_ w492]
          frame False {
          }
          frame True {
            n363 = invoke class="VI" method="Run VI"(reference=w492, "Wait until done"=FALSE ("结束前等待"), "Auto Dispose Ref"=FALSE ("自动销毁引用")) -> (reference out=w487:refnum<vi>)  [unwired: 2 in, 4 out]
            n364 = invoke class="VI" method="FP.Open"(reference=w487, "Activate"=TRUE ("激活？"), "State"=T14."Standard" ("状态")) -> ()  [unwired: 2 in, 5 out]
          }
        }
      }
      frame "Run top level" {
        n365 = case shown="假" w493 {
          tunnel: w494 -> [w495 _]
          frame False {
            n366 = invoke class="VI" method="Abort VI"(reference=w495) -> (reference out=w496:refnum<vi>)  [unwired: 2 in, 2 out]
            n367 = invoke class="VI" method="FP.Close"(reference=w496) -> ()  [unwired: 2 in, 3 out]
          }
          frame True {
          }
        }
      }
    }
    n368 = local write "运行模式"(w471) -> ()
    n369 = local write "时间阈值"(w469) -> ()
    n370 = local write "湿化学运行间隔"(w472) -> ()
    n371 = local write "周期设置"(w473) -> ()
    n372 = local write "流量阈值"(w470) -> ()
    n373 = local write "质控启动日期"(w476) -> ()
    n374 = local write "跨度核查时间"(w474) -> ()
    n375 = local write "自动运行启动参数"(w481) -> ()
    n376 = local write "空白核查时间"(w475) -> ()
    n377 = local write "24H周期设置"(w482) -> ()
    n378 = global read "系统设置全局变量.vi" "多参数运行间隔"() -> (w468:i16)
    n379 = local write "多参数运行间隔"(w468) -> ()
  }
  n380 = call <userlib>:"Abort Balloon Engine.vi"("error in (no error)"=w4, "SmartBalloon Engine Reference"=w5) -> ("error out"=w2:errorcluster)  [unwired: 9 in]
  n381 = call <vilib>:"Simple Error Handler.vi"("error in (no error)"=w2) -> ()  [unwired: 4 in, 5 out]
